vi "message_dialog_2.vi"(5 "(CANCEL) button text":string="CANCEL", 6 "name of caller in":string, 7 "(OK) button text":string="OK", 8 "Error in":errorcluster caption="Error in (no error)", 10 "flavour (error)":enum16{"error", "warning", "message"}(ring), 11 "text in":string="Undefined error occured.") -> (0 "Error out":errorcluster, 3 "ok?":bool)   [LabVIEW 2015]
panel:
  in  "ok":bool
  in  "cancel":bool
  out "text":string
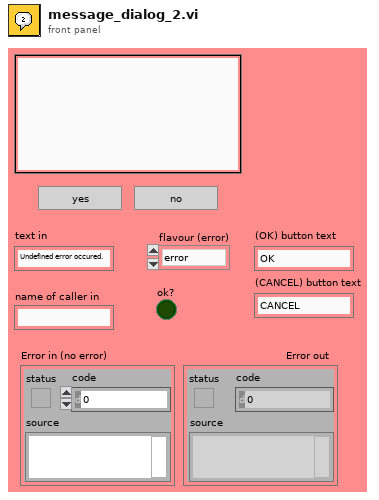
[diagram p1: front panel]
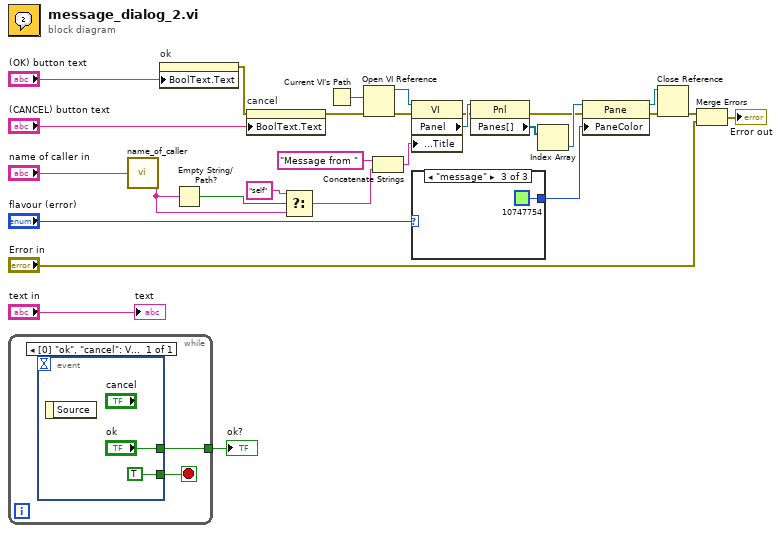
[diagram p0: block diagram]
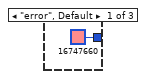
[diagram p2: hidden frame]
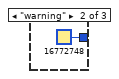
[diagram p3: hidden frame]
diagram:
  n1 = while {
    tunnel: [w29] -> w9
    stop <- w30 stop-if-true
    n2 = event shown="[0] \"ok\", \"cancel\": Value Change;  Panel Close;  Key Down" {
      selector: _ -> [_]
      dyn-events: _ -> [_]
      timeout: _ -> [_]
      tunnel: [TRUE] -> w30
      tunnel: ["ok"] -> w29
      event "ok", "cancel": Value Change; Panel Close; Key Down {
        n3 = event-data() -> ()  [unwired: 1 in, 1 out]
      }
    }
  }
  "ok?" <- w9
  n4 = call "name_of_caller.vi"("name of caller in"="name of caller in") -> ("name of caller out"=w13:string)  [unwired: 3 in]
  n5 = property on="ok" class="Bool"("BoolText.Text"="(OK) button text") -> (error out=w6:errorcluster)  [unwired: 2 in, 1 out]
  n6 = Empty String/Path?(string/path=w13) -> (empty?=w14:bool)
  n7 = property on="cancel" class="Bool"(error in=w6, "BoolText.Text"="(CANCEL) button text") -> (error out=w4:errorcluster)  [unwired: 1 in, 1 out]
  n8 = Select(t="self", s=w14, f=w13) -> (s? t:f=w12:string)
  n9 = Current VI's Path() -> (path=w28:path)
  n10 = Open VI Reference(vi path=w28, error in (no error)=w4) -> (vi reference=w27:refnum<vi>, error out=w17:errorcluster)  [unwired: 4 in]
  n11 = Concatenate Strings("Message from " ("string"), w12) -> (w15:string)
  n12 = property class="VI"(reference=w27, error in=w17, "Front Panel.Title"=w15) -> (error out=w18:errorcluster, "Panel"=w26:refnum<vi>)  [unwired: 1 out]
  n13 = case shown="\"message\"" "flavour (error)" {
    tunnel: [u32 16747660 u32 16772748 u32 10747754] -> w23
    frame "error", Default {
    }
    frame "warning" {
    }
    frame "message" {
    }
  }
  n14 = property class="Pnl"(reference=w26, error in=w18) -> (error out=w19:errorcluster, "Panes[]"=w25:refnum<vi>[])  [unwired: 1 out]
  n15 = Index Array(array=w25) -> (element=w22:refnum<vi>)  [unwired: 1 in]
  n16 = property class="Pane"(reference=w22, error in=w19, "PaneColor"=w23) -> (reference out=w21:refnum<vi>, error out=w20:errorcluster)
  n17 = Close Reference(reference=w21, error in (no error)=w20) -> (error out=w3:errorcluster)
  n18 = Merge Errors(w3, "Error in") -> (→"Error out":errorcluster)
  "text" <- "text in"
